vi "ModifyTestConfig.vi"(9 "TestItemsOut":refnum<vi>, 11 "Model":string) -> ()   [LabVIEW 2009]
uses:
  <vilib>/Utility/file.llb/Read From Spreadsheet File (string).vi
  <vilib>/Utility/file.llb/Write To Spreadsheet File (string).vi
panel:
  in  "CANCEL":bool
  in  "Save":bool
  in  "TestItems":string[][](table)
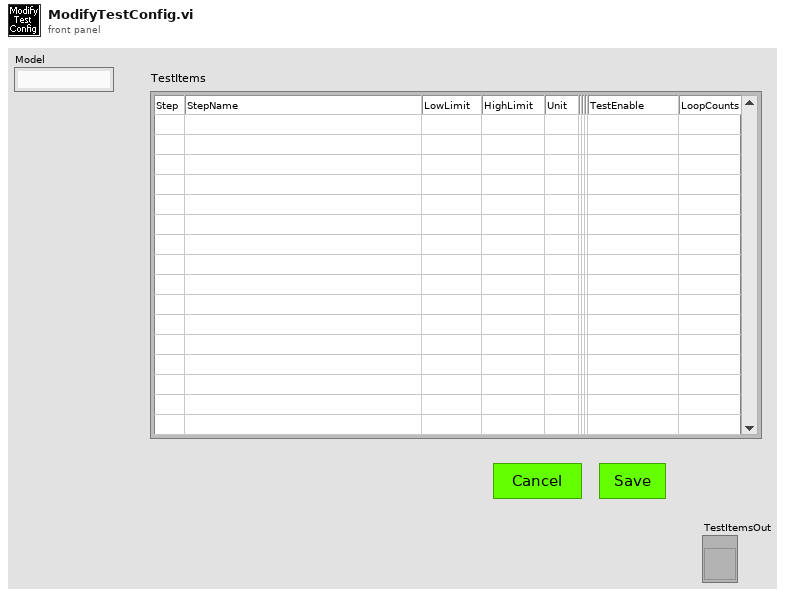
[diagram p1: front panel]
types:
  T1 = enum32{"invalid app kind", "Development System", "Run Time System", "Student Edition", "Embedded LabVIEW", "Evaluation", "Custom"}
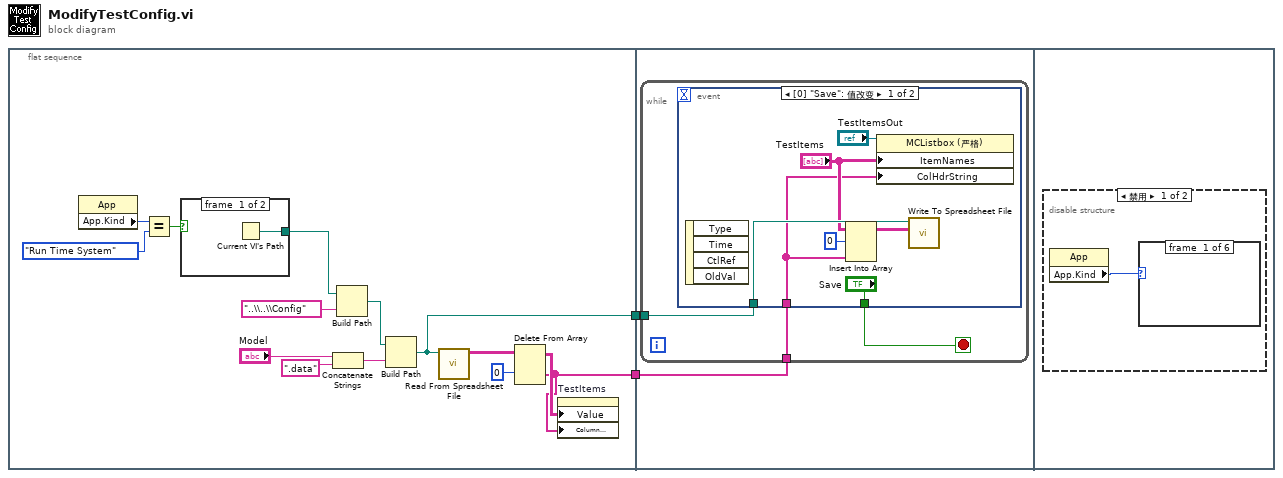
[diagram p0: block diagram]
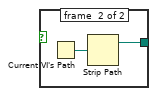
[diagram p2: hidden frame]
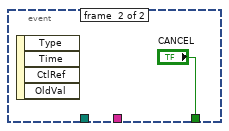
[diagram p3: hidden frame]
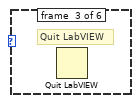
[diagram p5: hidden frame]
diagram:
  n1 = flat-sequence {
    tunnel: [w5] -> w2
    tunnel: [w3] -> w1
    tunnel: w2 -> [w21]
    tunnel: w1 -> [w20]
    frame #0 {
      n2 = property class="App"() -> ("App.Kind"=w13:T1)  [unwired: 2 in, 2 out]
      n3 = Equal?(x=w13, y=T1."Run Time System") -> (x = y?=w15:bool)
      n4 = case shown="真" w15 {
        tunnel: [w17 w19] -> w16
        frame #0 {
          n5 = Current VI's Path() -> (path=w17:path)
        }
        frame #1 {
          n6 = Current VI's Path() -> (path=w18:path)
          n7 = Strip Path(path=w18) -> (stripped path=w19:path)  [unwired: 1 out]
        }
      }
      n8 = Concatenate Strings("Model", ".data" ("pattern (all files)")) -> (w8:string)
      n9 = Build Path(base path=w16, name or relative path="..\\..\\Config" ("名称或相对路径")) -> (appended path=w11:path)
      n10 = Build Path(base path=w11, name or relative path=w8) -> (appended path=w5:path)
      n11 = call-poly <vilib>:"Read From Spreadsheet File.vi"("file path (dialog if empty)"=w5) -> ("all rows"=w6:string[][])  [unwired: 3 in, 7 out]
      n12 = Delete From Array(array=w6, index (row)=0 ("索引 (行)")) -> (deleted portion=w3:string[], array with subset deleted=w4:string[][])  [unwired: 2 in]
      n13 = property on="TestItems" class="Tbl (严格)"("Value"=w4, "Column Headers[]"=w3) -> ()  [unwired: 2 in, 2 out]
    }
    frame #1 {
      n14 = while {
        tunnel: w21 -> [w23]
        tunnel: w20 -> [w22]
        stop <- w24 stop-if-true
        n15 = event shown="[0] \"Save\": 值改变" {
          selector: _ -> [_ _]
          dyn-events: _ -> [_ _]
          timeout: _ -> [_ _]
          tunnel: ["Save" "CANCEL"] -> w24
          tunnel: w23 -> [w31 _]
          tunnel: w22 -> [w27 _]
          event #0 {
            n16 = event-data() -> ()  [unwired: 5 out]
            n17 = Insert Into Array(array="TestItems", index (row)=0 ("索引 (行)"), new element=w27) -> (w26:string[][])  [unwired: 1 in]
            n18 = property on="属性节点" class="MCListbox (严格)"(reference="TestItemsOut", "ItemNames"="TestItems", "ColHdrString"=w27) -> ()  [unwired: 1 in, 2 out]
            n19 = call-poly <vilib>:"Write To Spreadsheet File.vi"("2D data"=w26, "file path (dialog if empty)"=w31) -> ()  [unwired: 4 in, 3 out]
          }
          event #1 {
            n20 = event-data() -> ()  [unwired: 5 out]
          }
        }
      }
    }
    frame #2 {
      n21 = disable-structure shown="禁用" {
        frame #0 {
          n22 = property class="App"() -> ("App.Kind"=w33:T1)  [unwired: 2 in, 2 out]
          n23 = case shown="\"Run Time System\"" w33 {
            frame #0 {
            }
            frame #1 {
            }
            frame #2 {
              # "Quit LabVIEW"
              n24 = Quit LabVIEW() -> ()  [unwired: 1 in]
            }
            frame #3 {
            }
            frame #4 {
            }
            frame #5 {
            }
          }
        }
        frame #1 {
        }
      }
    }
  }
